vi "Alternating Number.vi"() -> ()   [LabVIEW 2016]
panel:
  out "Numeric":dbl
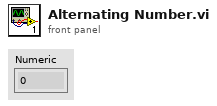
[diagram p1: front panel]
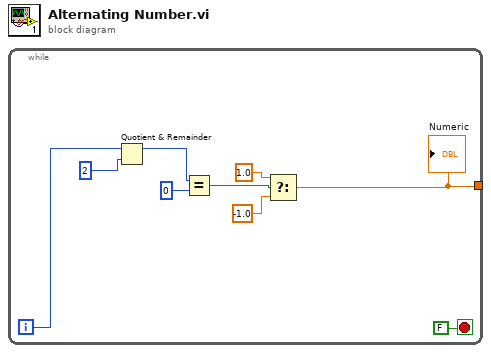
[diagram p0: block diagram]
diagram:
  n1 = while {
    tunnel: [w1] -> _
    i -> [w8]
    stop <- FALSE stop-if-true
    n2 = Quotient & Remainder(x=w8, y=2) -> (x-y*floor(x/y)=w7:i32)  [unwired: 1 out]
    n3 = Equal?(x=w7, y=0) -> (x = y?=w5:bool)
    n4 = Select(t=1.0, s=w5, f=-1.0) -> (s? t:f=w1:dbl)
    "Numeric" <- w1
  }
